vi "Trim Whitespace__ogtk.vi"   [LabVIEW 2011]
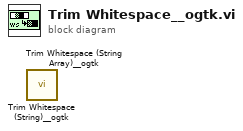
[diagram p0: block diagram]
diagram:
  n1 = call "Trim Whitespace (String)__ogtk.vi"() -> ()  [unwired: 7 in, 1 out]
  n2 = call "Trim Whitespace (String Array)__ogtk.vi"() -> ()  [unwired: 7 in, 1 out]
